vi "recharge.vi"() -> ()   [LabVIEW 2020]
panel:
  in  "PS error in":errorcluster caption="NHR error in (no error)"
  in  "Output Safety":T1
  in  "PS VISA in":refnum<visa-resource-name>
  out "data task out":refnum<k21>
  out "data task error out":errorcluster
  out "PS VIS resource name out":refnum<visa-resource-name>
  out "PS error out":errorcluster
  in  "Charge/Discharge\n time":dbl
  in  "Charge/Discharge Voltage Setpoint":dbl format="%#.6g"
  in  "Current Setpoint":dbl format="%#.6g"
  in  "Current Cutoff":dbl
  in  "data task error in":errorcluster
  in  "Data Task in":refnum<k21>
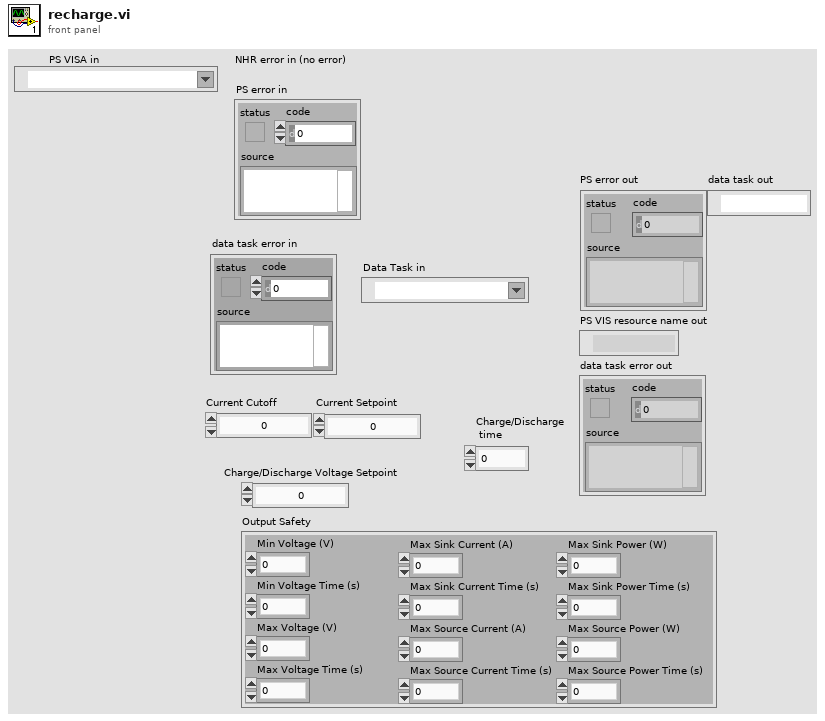
[diagram p1: front panel]
types:
  T1 = cluster{"Min Voltage (V)":dbl, "Min Voltage Time (s)":dbl, "Max Voltage (V)":dbl, "Max Voltage Time (s)":dbl, "Max Sink Current (A)":dbl, "Max Sink Current Time (s)":dbl, "Max Source Current (A)":dbl, "Max Source Current Time (s)":dbl, "Max Sink Power (W)":dbl, "Max Sink Power Time (s)":dbl, "Max Source Power (W)":dbl, "Max Source Power Time (s)":dbl}
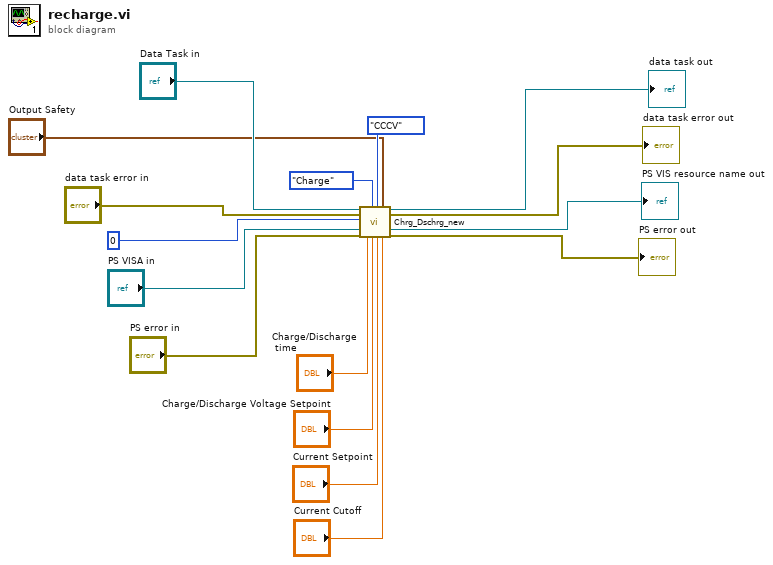
[diagram p0: block diagram]
diagram:
  n1 = call "Chrg_Dschrg_new.vi"("Data Task in"="Data Task in", "data task error in"="data task error in", "#DAQ outputs (1-13)"=0, "PS VISA in"="PS VISA in", "PS error in"="PS error in", "Charge/Discharge\n time"="Charge/Discharge\n time", "Charge/discharge"=enum8{"Charge", "Discharge"}."Charge", "Charge/Discharge Voltage Setpoint"="Charge/Discharge Voltage Setpoint", "CC or CCCV"=enum16{"CC", "CCCV"}."CCCV", "Current Setpoint"="Current Setpoint", "Output Safety"="Output Safety", "Current Cutoff"="Current Cutoff") -> ("data task out"=→"data task out":refnum<k21>, "data task error out"=→"data task error out":errorcluster, "PS VIS resource name out"=→"PS VIS resource name out":refnum<visa-resource-name>, "PS error out"=→"PS error out":errorcluster)  [unwired: 4 in]
